vi "Draw Disconnect Status.vi"(6 "Color Scheme":T1={"Black"=2302755, "Red"=16711695, "Green"=9232651, "Yellow"=16759040, "Blue"=36344, "Magenta"=7160742, "Cyan"=55531, "White"=15132390, "Bright Black"=4473924, "Bright Red"=16721728, "Bright Green"=11264347, "Bright Yellow"=16765506, "Bright Blue"=37631, "Bright Magenta"=10117099, "Bright Cyan"=6815728, "Bright White"=16777215}, 8 "Font":T2, 9 "Connected":bool, 10 "Draw Area Size":T3, 11 "Picture In":picture) -> (3 "Picture":picture)   [LabVIEW 2020, in "Terminal.lvlib" / "Terminal.lvclass"]
uses:
  Terminal.lvclass
  <vilib>/Utility/miscctls.llb/LVBoundsTypeDef.ctl
  Color Scheme.ctl
  Terminal.lvclass/Terminal.ctl
  Terminal.lvlib
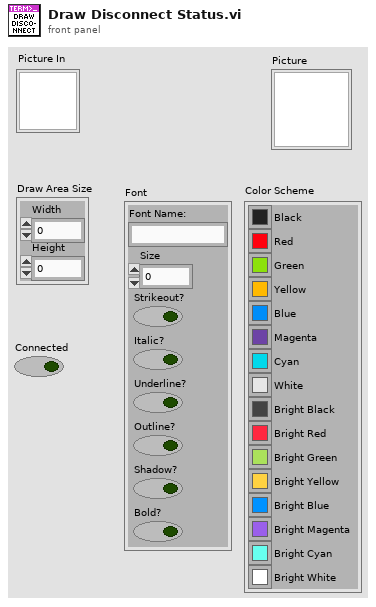
[diagram p1: front panel]
types:
  T1 = typedef "Terminal.lvlib/Color Scheme.ctl" = cluster{"Black":u32, "Red":u32, "Green":u32, "Yellow":u32, "Blue":u32, "Magenta":u32, "Cyan":u32, "White":u32, "Bright Black":u32, "Bright Red":u32, "Bright Green":u32, "Bright Yellow":u32, "Bright Blue":u32, "Bright Magenta":u32, "Bright Cyan":u32, "Bright White":u32}
  T2 = cluster{"Font Name:":string, "Size":i16, "Strikeout?":bool, "Italic?":bool, "Underline?":bool, "Outline?":bool, "Shadow?":bool, "Bold?":bool}
  T3 = typedef "LVBoundsTypeDef.ctl" = cluster{"Width":u32, "Height":u32}
  T4 = cluster{"left":i16, "top":i16, "right":i16, "bottom":i16}
  T5 = enum16{"User-specified Font", "Application Font", "System Font", "Dialog Font"}
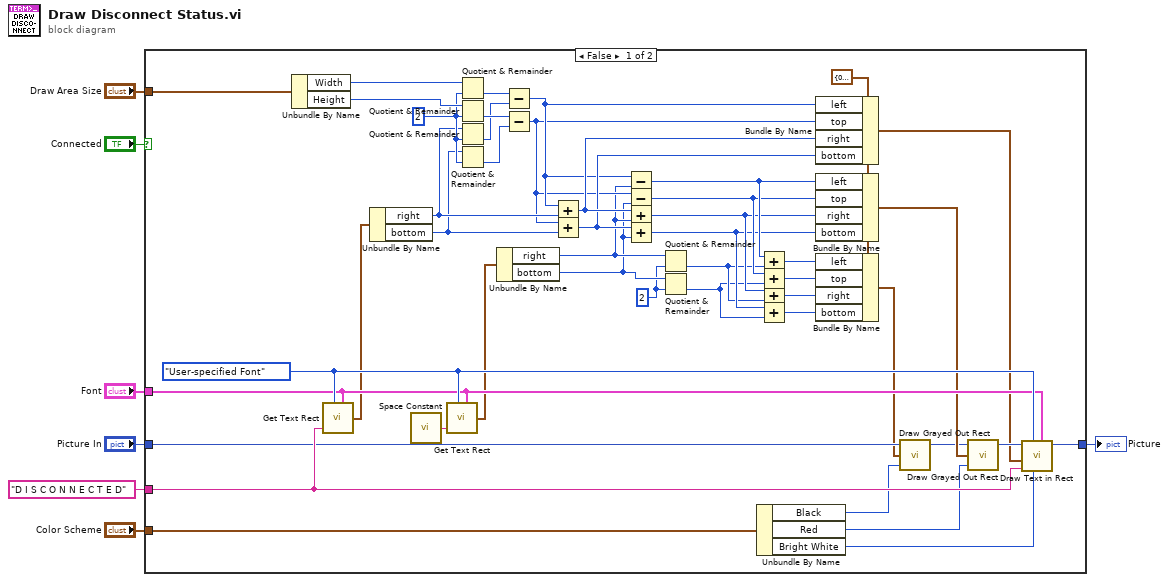
[diagram p0: block diagram]
diagram:
  n1 = case shown="False" "Connected" {
    tunnel: [w46 w53] -> w2
    tunnel: "Font" -> [w51 _]
    tunnel: "D I S C O N N E C T E D" ("text") -> [w37 _]
    tunnel: "Draw Area Size" -> [w29 _]
    tunnel: "Picture In" -> [w27 w53]
    tunnel: "Color Scheme" -> [w11 _]
    frame False {
      w14 = i16 2 ("y")
      w42 = i16 2 ("y")
      w26 = T4 {"left"=0, "top"=0, "right"=0, "bottom"=0} ("rect")
      w52 = T5."User-specified Font" ("desired font(Application)")
      n2 = Unbundle By Name(w29) -> ("Width"=w43:u32, "Height"=w44:u32)
      n3 = call <vilib>:"Get Text Rect.vi"("desired font(Application)"=w52, "text"=w37, "[user-specified font]"=w51) -> ("rect"=w48:T4)  [unwired: 6 in]
      n4 = Unbundle By Name(w48) -> ("right"=w32:i16, "bottom"=w31:i16)
      n5 = call <vilib>:"Space Constant.vi"() -> ("String"=w50:string)
      n6 = call <vilib>:"Get Text Rect.vi"("desired font(Application)"=w52, "text"=w50, "[user-specified font]"=w51) -> ("rect"=w49:T4)  [unwired: 6 in]
      n7 = Quotient & Remainder(x=w43, y=w42) -> (floor(x/y)=w41:u32)  [unwired: 1 out]
      n8 = Quotient & Remainder(x=w44, y=w42) -> (floor(x/y)=w40:u32)  [unwired: 1 out]
      n9 = Quotient & Remainder(x=w32, y=w42) -> (floor(x/y)=w39:i16)  [unwired: 1 out]
      n10 = Quotient & Remainder(x=w31, y=w42) -> (floor(x/y)=w38:i16)  [unwired: 1 out]
      n11 = Unbundle By Name(w49) -> ("right"=w16:i16, "bottom"=w15:i16)
      n12 = Subtract(x=w41, y=w39) -> (x-y=w33:u32)
      n13 = Subtract(x=w40, y=w38) -> (x-y=w30:u32)
      n14 = Add(x=w33, y=w32) -> (x+y=w35:u32)
      n15 = Add(x=w30, y=w31) -> (x+y=w34:u32)
      n16 = Subtract(x=w33, y=w16) -> (x-y=w20:u32)
      n17 = Subtract(x=w30, y=w15) -> (x-y=w19:u32)
      n18 = Add(x=w35, y=w16) -> (x+y=w18:u32)
      n19 = Add(x=w34, y=w15) -> (x+y=w17:u32)
      n20 = Quotient & Remainder(x=w16, y=w14) -> (floor(x/y)=w13:i16)  [unwired: 1 out]
      n21 = Quotient & Remainder(x=w15, y=w14) -> (floor(x/y)=w12:i16)  [unwired: 1 out]
      n22 = Unbundle By Name(w11) -> ("Black"=w10:u32, "Red"=w9:u32, "Bright White"=w8:u32)
      n23 = Add(x=w20, y=w13) -> (x+y=w24:u32)
      n24 = Add(x=w19, y=w12) -> (x+y=w21:u32)
      n25 = Add(x=w18, y=w13) -> (x+y=w23:u32)
      n26 = Add(x=w17, y=w12) -> (x+y=w22:u32)
      n27 = Bundle By Name(cluster=w26, "left"=w33, "top"=w30, "right"=w35, "bottom"=w34) -> (w36:T4)
      n28 = Bundle By Name(cluster=w26, "left"=w20, "top"=w19, "right"=w18, "bottom"=w17) -> (w45:T4)
      n29 = Bundle By Name(cluster=w26, "left"=w24, "top"=w21, "right"=w23, "bottom"=w22) -> (w25:T4)
      n30 = call <vilib>:"Draw Grayed Out Rect.vi"("color(black)"=w10, "rect"=w25, "picture"=w27) -> ("new picture"=w28:picture)  [unwired: 2 in]
      n31 = call <vilib>:"Draw Grayed Out Rect.vi"("color(black)"=w9, "rect"=w45, "picture"=w28) -> ("new picture"=w47:picture)  [unwired: 2 in]
      n32 = call <vilib>:"Draw Text in Rect.vi"("[user-specified font]"=w51, "text color(black)"=w8, "desired font(Application)"=w52, "text"=w37, "rect"=w36, "picture"=w47) -> ("new picture"=w46:picture)  [unwired: 5 in]
    }
    frame True {
    }
  }
  "Picture" <- w2
